vi "SpeakerTaskVocalizations.vi"(0 "stop":bool, 2 "Physical Channels":tag="Dev1/ao0:1", 5 "String":string) -> (1 "Waveform Graph":waveform(dbl)(graph)={"t0"=timestamp(0 s since 1904-01-01), "dt"=6.25e-05, "Y"=[9.1552734375e-05]})   [LabVIEW 2010]
doc: "I. Description:\nThis example demonstrates how to output a continuous periodic waveform using an internal sample clock.\n\nII. Instructions for Running:\n1. Select the Physical Channel to correspond to where your signal is output on the DAQ device.\n2. Enter the Minimum and Maximum Voltage Ranges\n3. Specify the Desired Frequency of the output Waveform\n4. Enter the Waveform Information. See the documentation of the Waveform Buffer Generation SubVI for information on each parameter.\n\nIII. Block Diagram Steps:\n1. Create an Analog Output Voltage channel.\n2. Call the DAQmx Timing (Use Waveform) VI which sets the sample clock rate based on the input waveform parameters, and set the sample mode to Continuous.\n3. Write the waveform to the output buffer.\n4. Call the Start VI.\n5. Loop continuously until the user presses the Stop button. Check for errors every 100 ms using the Is Task Done? VI\n6. Clear the Task\n7. Use the popup dialog box to display an error or warning if any.\n\nIV. I/O Connections Overview:\nMake sure your signal output terminal matches the Physical Channel I/O Control. For further connection information, refer to your hardware reference manual."
uses:
  <vilib>/Utility/error.llb/DialogType.ctl
  <vilib>/DAQmx/write.llb/DAQmx Write (Analog 1D DBL 1Chan NSamp).vi
  <vilib>/DAQmx/create/channels.llb/DAQmx Create Channel (AO-Voltage-Basic).vi
  <vilib>/DAQmx/configure/timing.llb/DAQmx Timing (Sample Clock).vi
  <vilib>/imath/engines/lvmath2/RunTimeEngine/ErrorHandling/NIMS_Finalize Error.vi
  <vilib>/imath/engines/lvmath2/RunTimeEngine/Managers/WorkSpace/UID Generator.vi
  <vilib>/imath/engines/lvmath/Plug In/_Char/NIMS_CH_String to Character Array.vi
  <vilib>/imath/engines/lvmath2/RunTimeEngine/Managers/SymbolTable/Clear UID.vi
  <vilib>/imath/engines/lvmath2/RunTimeEngine/NodeEndStatement/NIMS_NodeEndStatement_Output.vi
  <instcachedir>/0/NIMS_NodeEndStatement_Output_53EC0D466D134D7ABD903AC30B43404B.lvgen/NIMS_NodeEndStatement_Output_53EC0D466D134D7ABD903AC30B43404B_001.vi
  <instcachedir>/0/NIMS_NodeEndStatement_Output_53EC0D466D134D7ABD903AC30B43404B.lvgen/NIMS_NodeEndStatement_Output_53EC0D466D134D7ABD903AC30B43404B_002.vi
  <vilib>/imath/engines/lvmath/Plug In/_Char/NIMS_CH_Character RV to String.vi
  <vilib>/imath/engines/lvmath2/RunTimeEngine/BuiltInFunctions/wavread/NIMS_wavread(Str,I32V).vi
  <vilib>/imath/engines/lvmath2/RunTimeEngine/RunTimeType/NIMS_RunTimeType_From StrictType (excl LVString).vi
  <vilib>/imath/engines/lvmath2/RunTimeEngine/LocalVariableDefStatement/MC_LocalVariableDefStatement_Display.vi
  <vilib>/measure/maspectr.llb/FFT Power Spectrum for 1 Chan.vi
  <vilib>/daqmx/miscellaneous.llb/DAQmx Fill In Error Info.vi
  <vilib>/measure/NI_MAPro.lvlib
  <vilib>/imath/engines/lvmath2/RunTimeEngine/Managers/SymbolTable/NIMS_WorkSpace.lvlib
panel:
  in  "Power Spectrum":bool
  out "Power Spectrum 2":cluster{"f0":dbl, "df":dbl, "magnitude":dbl[]}(graph)={"f0"=0.0, "df"=0.19999909297463503, "magnitude"=array[110251 elements]}
  out "Done":bool=TRUE
  out "Completed":dbl=1.0 format="%0.0f"
  in  "restart":bool
  in  "dB":bool=TRUE
  in  "stop 2":bool
  in  "window":T1(ring)=enum."Hanning"
  in  "averaging parameters":T2={"averaging mode"=enum."No averaging", "weighting mode"=enum."Exponential", "number of averages"=10} {"number of averages" min=1}
  in  "Minimum Value":dbl=-10.0 format="%0.2f"
  in  "Maximum Value":dbl=10.0 format="%0.2f"
  # "Real-Time Spectral Measurements"
  # "Sampling Rate"
  # "Wav File"
  # "Channel Parameters"
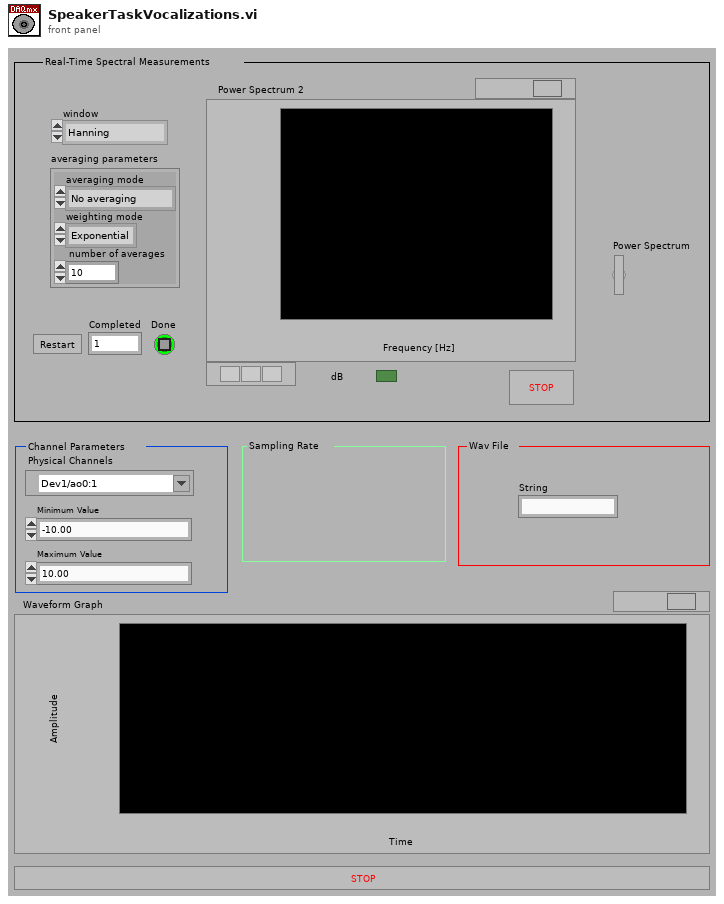
[diagram p1: front panel]
types:
  T1 = enum16{"None ", "Hanning", "Hamming", "Blackman-Harris", "Exact Blackman", "Blackman", "Flat Top", "4 Term B-Harris ", "7 Term B-Harris", "Low Sidelobe"}
  T2 = cluster{"averaging mode":enum16{"No averaging", "Vector averaging", "RMS averaging", "Peak hold"}, "weighting mode":enum16{"Linear", "Exponential"}, "number of averages":u32}
  T3 = typedef "DialogType.ctl" = u16
  T4 = enum16{"Initialize", "String", "Start", "New Session", "Stop", "Resume", "Close"}
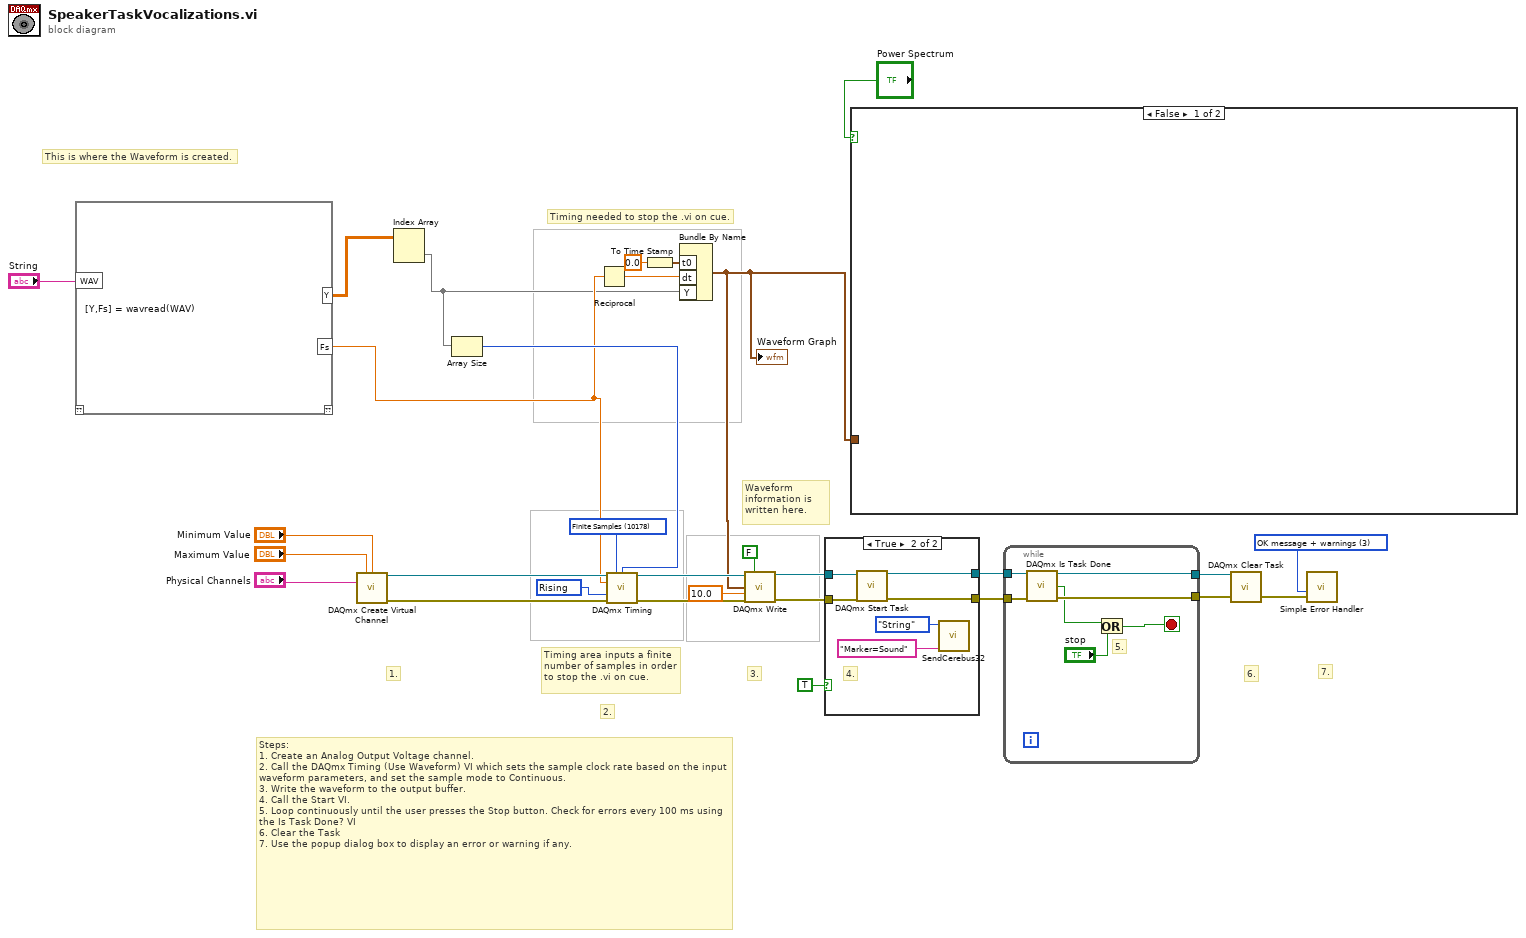
[diagram p0: block diagram]
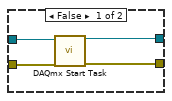
[diagram p2: hidden frame]
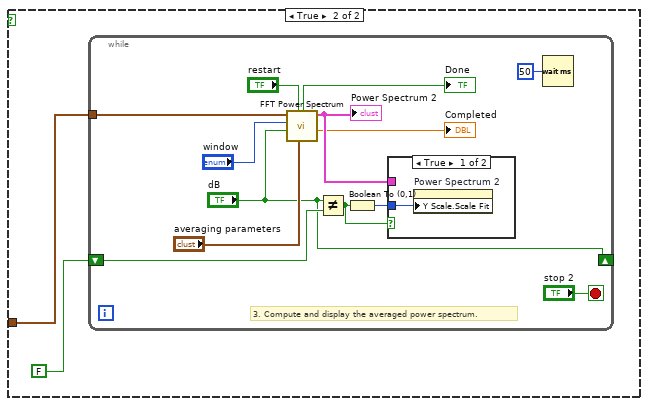
[diagram p3: hidden frame]
diagram:
  w13 = 10280 items=["Rising"=10280, "Falling"=10171] ("active edge")
  w18 = T3 3 items=["no dialog", "OK message", "continue or stop message", "OK message + warnings", "continue/stop + warnings"] ("type of dialog (OK msg:1)")
  w29 = 10178 items=["Finite Samples"=10178, "Continuous Samples"=10123] ("sample mode")
  # "Waveform information is written here."
  # "Timing area inputs a finite number of samples in order to stop the .vi on cue."
  # "Timing needed to stop the .vi on cue."
  # "This is where the Waveform is created."
  # "7."
  # "6."
  # "Steps: \n1. Create an Analog Output Voltage channel.\n2. Call the DAQmx Timing (Use Waveform) VI which sets the sample clock rate based on the input waveform parameters, and set the sample mode to Continuous.\n3. Write the waveform to the output buffer.\n4. Call the Start VI.\n5. Loop continuously until the user presses the Stop button. Check for errors every 100 ms using the Is Task Done? VI\n6. Clear the Task\n7. Use the popup dialog box to display an error or warning if any."
  # "3."
  # "2."
  # "1."
  n1 = mathscript code="[Y,Fs] = wavread(WAV)"("WAV"="String") -> ("Y"=w3:dbl[][], "Fs"=w4:dbl)  [unwired: 1 in, 1 out]
  n2 = call-poly <vilib>:"DAQmx Create Virtual Channel.vi"("maximum value"="Maximum Value", "minimum value"="Minimum Value", "physical channels"="Physical Channels") -> ("task out"=w15:refnum<k21>, "error out"=w14:errorcluster)  [unwired: 11 in]
  n3 = Index Array(array=w3) -> (element=w2:dbl[])  [unwired: 2 in]
  n4 = Array Size(array=w2) -> (size(s)=w7:i32)
  n5 = Reciprocal(x=w4) -> (1/x=w10:dbl)
  n6 = call-poly <vilib>:"DAQmx Timing.vi"("task/channels in"=w15, "sample mode"=w29, "samples per channel"=w7, "rate"=w4, "active edge"=w13, "error in"=w14) -> ("task out"=w21:refnum<k21>, "error out"=w20:errorcluster)  [unwired: 8 in]
  n7 = To Time Stamp(1:0.0 ("number")) -> (0:w12:timestamp)
  n8 = Bundle By Name("t0"=w12, "dt"=w10, "Y"=w2) -> (w1:waveform(dbl))  [unwired: 1 in]
  "Waveform Graph" <- w1
  n9 = call-poly <vilib>:"DAQmx Write.vi"("task/channels in"=w21, "auto start"=FALSE, "data"=w1, "timeout"=10.0 ("Wirite Timeout"), "error in"=w20) -> ("task out"=w26:refnum<k21>, "error out"=w25:errorcluster)  [unwired: 8 in, 1 out]
  n10 = case shown="True" TRUE {
    tunnel: w26 -> [w34 w40]
    tunnel: w25 -> [w33 w39]
    tunnel: [w31 w38] -> w23
    tunnel: [w32 w37] -> w19
    frame False {
      n11 = call <vilib>:"DAQmx Start Task.vi"("task/channels in"=w34, "error in"=w33) -> ("task out"=w32:refnum<k21>, "error out"=w31:errorcluster)  [unwired: 12 in]
    }
    frame True {
      # "4."
      n12 = call <vilib>:"DAQmx Start Task.vi"("task/channels in"=w40, "error in"=w39) -> ("task out"=w37:refnum<k21>, "error out"=w38:errorcluster)  [unwired: 12 in]
      n13 = call "SendCerebus32.vi"("String"="Marker=Sound" ("ASCII Data"), "Mode"=T4."String") -> ()  [unwired: 3 in]
    }
  }
  n14 = case shown="False" "Power Spectrum" {
    tunnel: w1 -> [_ w41]
    frame False {
    }
    frame True {
      n15 = while {
        shift-left: FALSE ("dB") -> [w49]
        shift-right: ["dB"] -> _
        tunnel: w41 -> [w43]
        stop <- "stop 2" stop-if-true
        # "3. Compute and display the averaged power spectrum."
        n16 = call-poly <vilib>:"FFT Power Spectrum.vi"("averaging parameters"="averaging parameters", "restart averaging (F)"="restart", "dB On (F)"="dB", "window"="window", "time signal"=w43) -> ("averages completed"=→"Completed":dbl, "power spectrum"=w53:cluster{"f0":dbl, "df":dbl, "magnitude":dbl[]}, "averaging done"=→"Done":bool)  [unwired: 3 in, 1 out]
        "Power Spectrum 2" <- w53
        n17 = Not Equal?(x="dB", y=w49) -> (x != y?=w48:bool)
        n18 = Boolean To (0,1)(Boolean=w48) -> (0, 1=w47:i16)
        n19 = case shown="True" w48 {
          tunnel: w47 -> [w56 _]
          tunnel: w53 -> [_ _]
          frame True {
            n20 = property on="Power Spectrum 2" class="WFGraph (strict)"("Y Scale.Scale Fit"=w56) -> ()  [unwired: 2 in, 2 out]
          }
          frame False {
          }
        }
        n21 = Wait (ms)(milliseconds to wait=u32 50 ("millisecond multiple")) -> ()  [unwired: 1 out]
      }
    }
  }
  n22 = while {
    tunnel: w19 -> [w63]
    tunnel: [w62] -> w17
    tunnel: w23 -> [w61]
    tunnel: [w60] -> w16
    stop <- w59 stop-if-true
    # "5."
    n23 = call <vilib>:"DAQmx Is Task Done.vi"("task/channels in"=w63, "error in"=w61) -> ("task out"=w62:refnum<k21>, "task done?"=w57:bool, "error out"=w60:errorcluster)  [unwired: 11 in]
    n24 = Or(x=w57, y="stop") -> (x .or. y?=w59:bool)
  }
  n25 = call <vilib>:"DAQmx Clear Task.vi"("task in"=w17, "error in"=w16) -> ("error out"=w30:errorcluster)  [unwired: 13 in]
  n26 = call <vilib>:"Simple Error Handler.vi"("type of dialog (OK msg:1)"=w18, "error in (no error)"=w30) -> ()  [unwired: 3 in, 5 out]
